vi "继保.vi"() -> ()   [LabVIEW 2015]
uses:
  <vilib>/Modbus/master/Modbus Master.lvclass
  <userlib>/QMH/Message Queue/Support/Enqueue Message (Single).vi
  Global control/global-2.vi
  <vilib>/Modbus/master/Create Master Instance (TCP).vi
  <userlib>/QMH/User Event - Stop/User Event - Stop.lvlib
  <userlib>/QMH/Message Queue/Message Queue.lvlib
panel:
  out "开入":T1
  out "软压板R":T2 caption="继保遥信"
  out "动作报告":T3
  out "虚遥信":T4
  in  "软压板W":T2 caption="继保遥信"
  in  "遥控1合":bool
  in  "遥控1分":bool
  out "遥控R":bool[](array[boolean])
  in  "HostThread":variant
  in  "Exit":bool
  out "遥测":u32[](array[numeric])
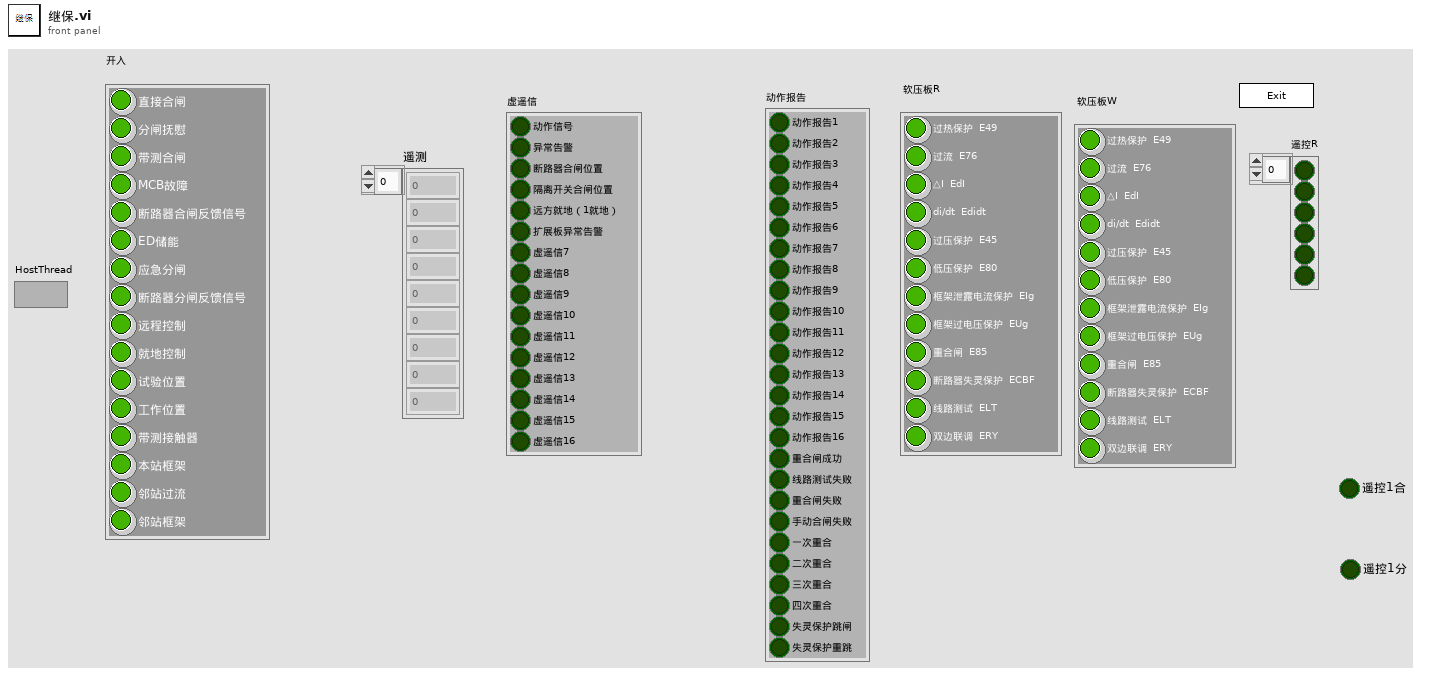
[diagram p1: front panel]
types:
  T1 = cluster{"直接合闸":bool, "分闸抚慰":bool, "带测合闸":bool, "MCB故障":bool, "断路器合闸反馈信号":bool, "ED储能":bool, "应急分闸":bool, "断路器分闸反馈信号":bool, "远程控制":bool, "就地控制":bool, "试验位置":bool, "工作位置":bool, "带测接触器":bool, "本站框架":bool, "邻站过流":bool, "邻站框架":bool}
  T2 = cluster{"过热保护  E49":bool, "过流  E76":bool, "△I  EdI":bool, "di/dt  Edidt":bool, "过压保护  E45":bool, "低压保护  E80":bool, "框架泄露电流保护  EIg":bool, "框架过电压保护  EUg":bool, "重合闸  E85":bool, "断路器失灵保护  ECBF":bool, "线路测试  ELT":bool, "双边联调  ERY":bool}
  T3 = cluster{"动作报告1":bool, "动作报告2":bool, "动作报告3":bool, "动作报告4":bool, "动作报告5":bool, "动作报告6":bool, "动作报告7":bool, "动作报告8":bool, "动作报告9":bool, "动作报告10":bool, "动作报告11":bool, "动作报告12":bool, "动作报告13":bool, "动作报告14":bool, "动作报告15":bool, "动作报告16":bool, "重合闸成功":bool, "线路测试失败":bool, "重合闸失败":bool, "手动合闸失败":bool, "一次重合":bool, "二次重合":bool, "三次重合":bool, "四次重合":bool, "失灵保护跳闸":bool, "失灵保护重跳":bool}
  T4 = cluster{"动作信号":bool, "异常告警":bool, "断路器合闸位置":bool, "隔离开关合闸位置":bool, "远方就地（1就地）":bool, "扩展板异常告警":bool, "虚遥信7":bool, "虚遥信8":bool, "虚遥信9":bool, "虚遥信10":bool, "虚遥信11":bool, "虚遥信12":bool, "虚遥信13":bool, "虚遥信14":bool, "虚遥信15":bool, "虚遥信16":bool}
  T5 = cluster{"Controls":cluster{"Exit":refnum<vi>}, "Thread":cluster{"ThisQ":string, "ThisVI":refnum<vi>, "HostQ":string, "HostRef":refnum<vi>, "SlavesQ":string[], "SlavesRef":refnum<vi>[]}, "Data":cluster{"Replace":bool}, "User":cluster{"Name":string}, "TCP master instance":refnum<class "Modbus Master.lvclass">}
  T6 = cluster{"开入1":bool, "开入2":bool, "开入3":bool, "开入4":bool, "开入5":bool, "开入6":bool, "开入7":bool, "开入8":bool, "开入9":bool, "开入10":bool, "开入11":bool, "开入12":bool, "开入13":bool, "开入14":bool, "开入15":bool, "开入16":bool}
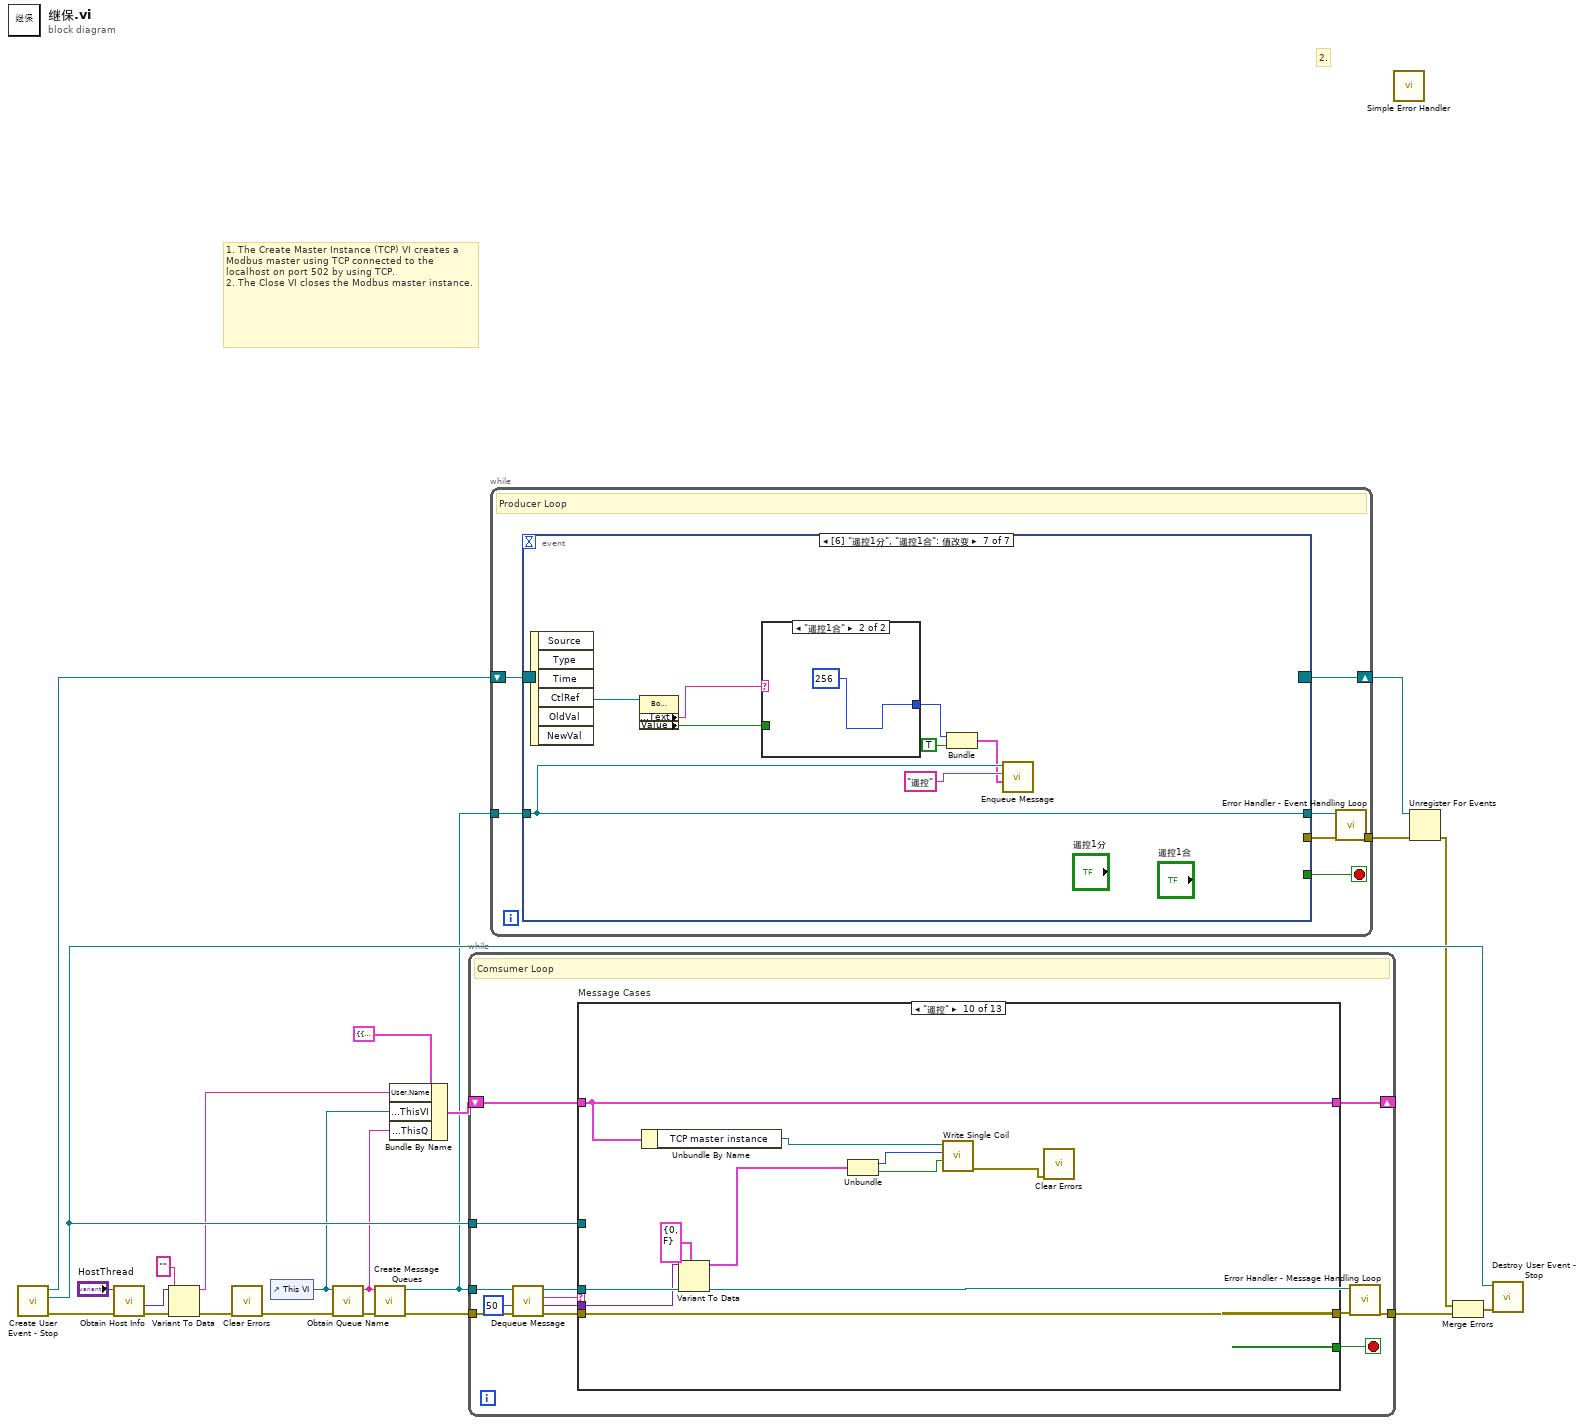
[diagram p0: block diagram]
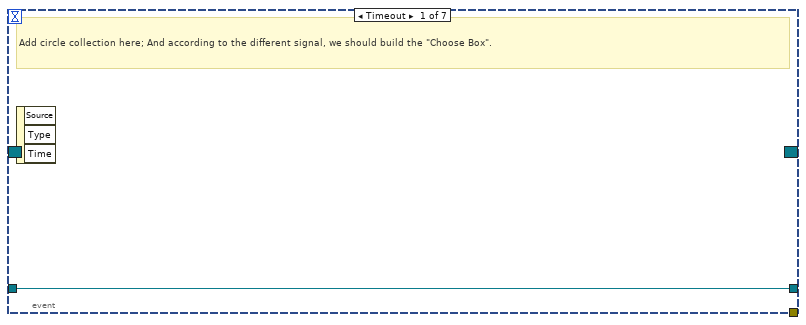
[diagram p2: hidden frame]
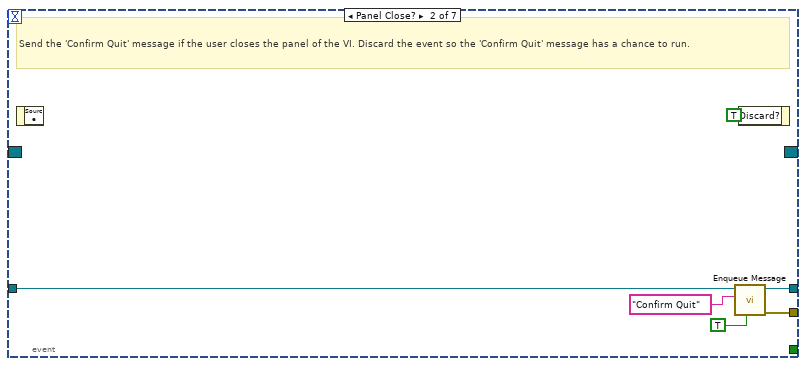
[diagram p3: hidden frame]
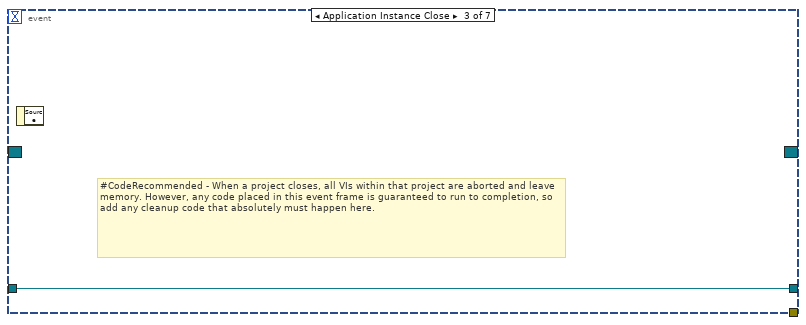
[diagram p4: hidden frame]
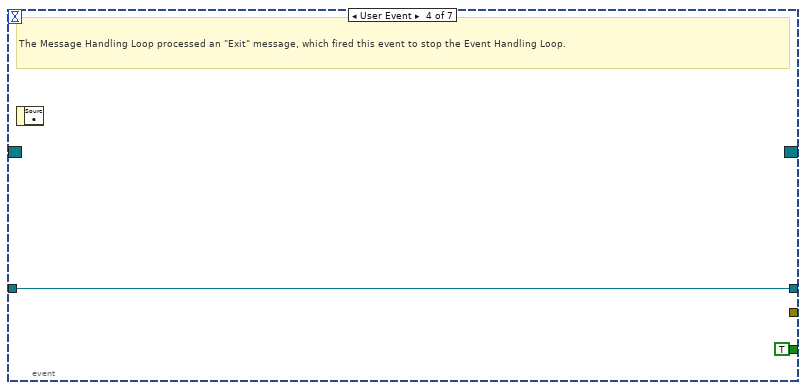
[diagram p5: hidden frame]
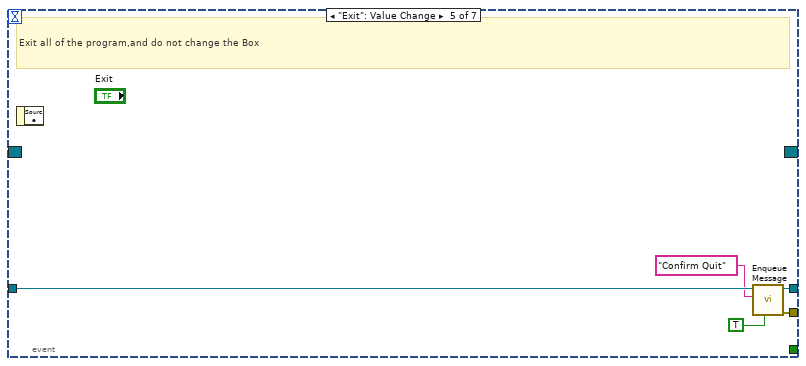
[diagram p6: hidden frame]
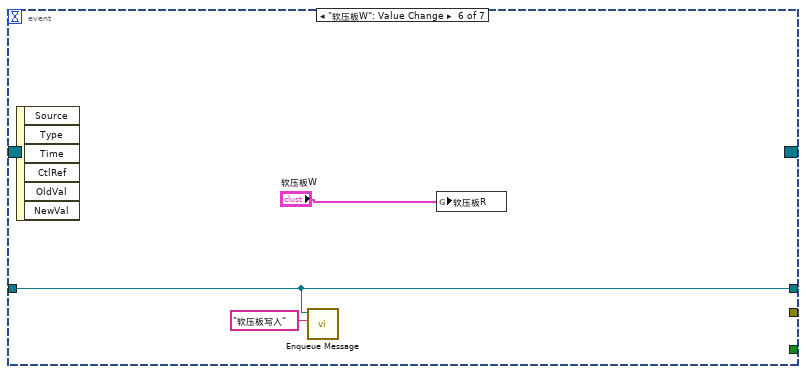
[diagram p7: hidden frame]
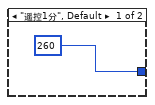
[diagram p8: hidden frame]
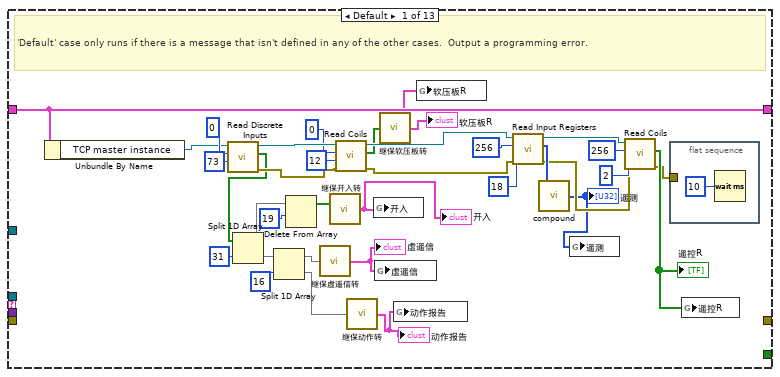
[diagram p9: hidden frame]
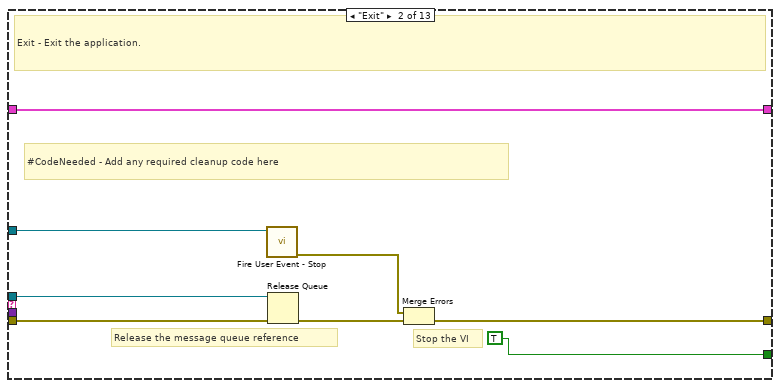
[diagram p10: hidden frame]
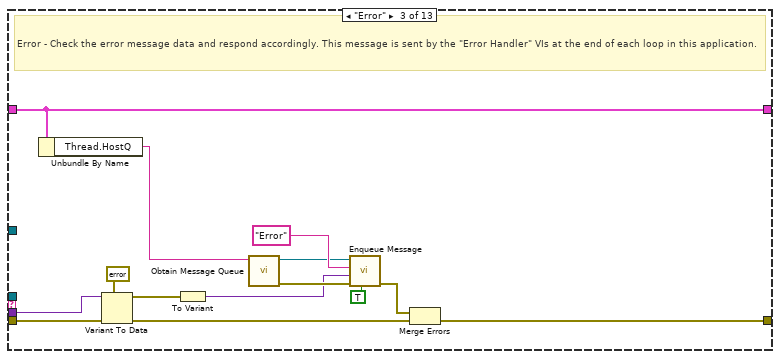
[diagram p11: hidden frame]
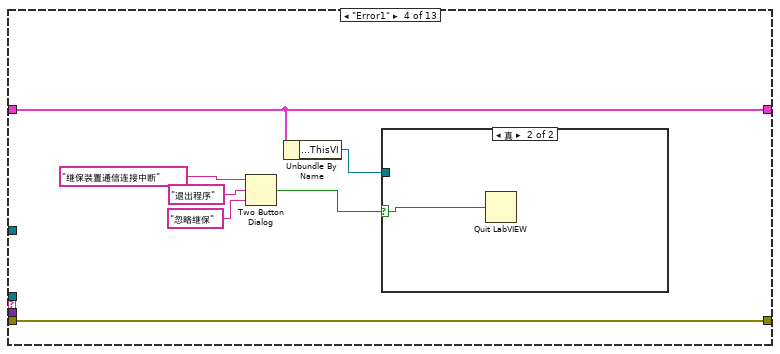
[diagram p12: hidden frame]
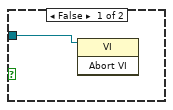
[diagram p13: hidden frame]
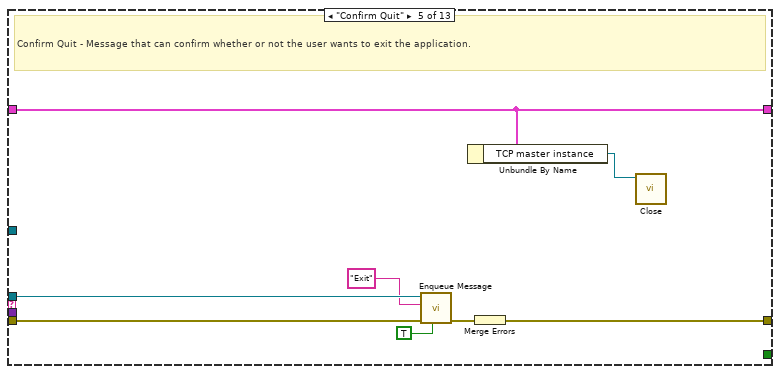
[diagram p14: hidden frame]
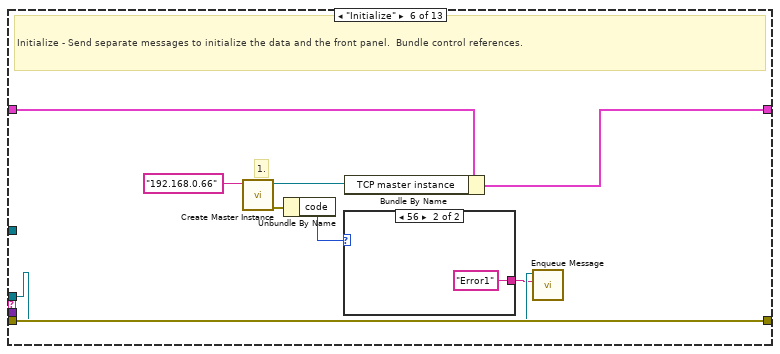
[diagram p15: hidden frame]
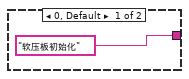
[diagram p16: hidden frame]
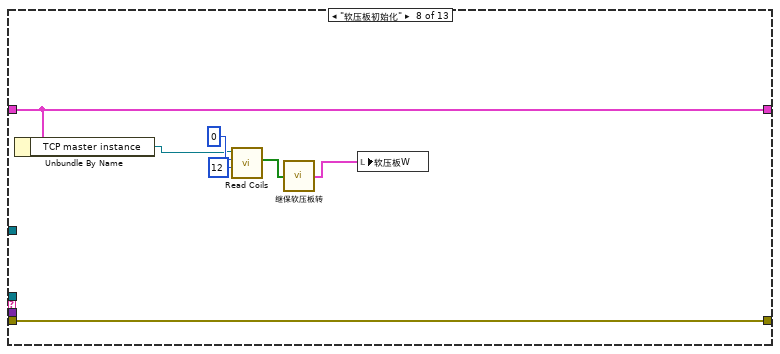
[diagram p18: hidden frame]
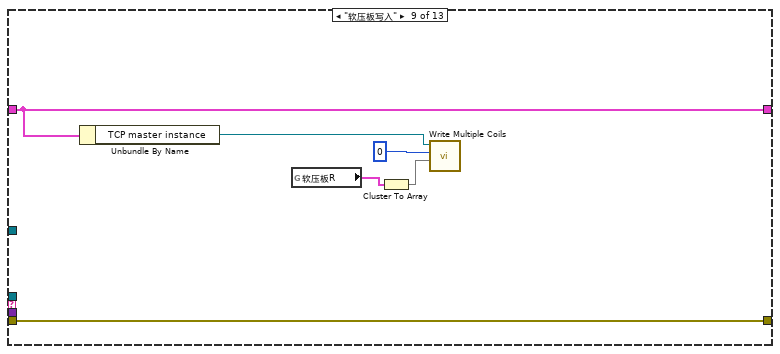
[diagram p19: hidden frame]
diagram:
  # "2."
  # "1. The Create Master Instance (TCP) VI creates a Modbus master using TCP connected to the localhost on port 502 by using TCP.\n2. The Close VI closes the Modbus master instance."
  n1 = call <userlib>:"Create User Event - Stop.vi"() -> ("error out"=w9:errorcluster, "User Event - Stop"=w18:refnum<user-event>, "Stop Event Registration Refnum"=w20:refnum<event-registration>)  [unwired: 9 in]
  n2 = call <userlib>:"Obtain Host Info.vi"("error in (no error)"=w9, "HostThread"="HostThread") -> ("error out"=w6:errorcluster, "Data"=w5:variant)  [unwired: 6 in, 2 out]
  n3 = Variant To Data(error in=w6, type="", Variant=w5) -> (data=w1:string, error out=w3:errorcluster)
  n4 = call <vilib>:"Clear Errors.vi"("error in (no error)"=w3) -> ("error out"=w2:errorcluster)  [unwired: 5 in, 1 out]
  n5 = control-ref of="This VI"() -> (w11:refnum<vi>)
  n6 = call <userlib>:"Obtain Queue Name.vi"("error in (no error)"=w2, "VI Refnum"=w11) -> ("error out"=w14:errorcluster, "ViName"=w10:string)  [unwired: 8 in]
  n7 = call <userlib>:"Create Message Queues.vi"("error in (no error)"=w14, "name (unnamed)"=w10) -> ("error out"=w22:errorcluster, "QueueHandler"=w7:refnum<queue>)  [unwired: 8 in]
  n8 = Bundle By Name(cluster=T5 {"Controls"={"Exit"=refnum}, "Thread"={"ThisQ"="", "ThisVI"=refnum, "HostQ"="", "HostRef"=refnum, "SlavesQ"=[], "SlavesRef"=[]}, "Data"={"Replace"=FALSE}, "User"={"Name"=""}, "TCP master instance"=refnum} ("Data Cluster"), "User.Name"=w1, "Thread.ThisVI"=w11, "Thread.ThisQ"=w10) -> (w12:T5)
  n9 = while {
    tunnel: w7 -> [w27]
    shift-right: [w34] -> _
    shift-left: w12 -> [w35]
    tunnel: w18 -> [w32]
    tunnel: w22 -> [w31]
    tunnel: [w25] -> w21
    stop <- w33 stop-if-true
    # "Comsumer Loop"
    n10 = call <userlib>:"Dequeue Message.vi"("error in (no error)"=w31, "timeout in ms (-1)"=50, "Message Queue"=w27) -> ("error out"=w30:errorcluster, "Message Data"=w28:variant, "Message"=w29:string, "dup Message Queue"=w26:refnum<queue>)  [unwired: 5 in]
    n11 = case "Message Cases" shown="\"遥控\"" w29 {
      tunnel: w26 -> [_ w78 _ _ w106 w111 _ _ _ _ _ _ _]
      tunnel: w30 -> [_ w73 w92 w99 w109 w118 w122 w129 w135 w144 w146 w147 w150]
      tunnel: [_ w74 w87 w99 w108 w118 w122 w129 w135 w144 w146 w147 w150] -> w24
      tunnel: w35 -> [w58 w77 w84 w94 w103 w116 w121 w126 w134 w143 w145 w148 w149]
      tunnel: [w58 w77 w84 w94 w103 w115 w121 w126 w134 w143 w145 w148 w149] -> w34
      tunnel: [_ TRUE _ _ _ _ _ _ _ _ _ _ _] -> w33
      tunnel: w28 -> [_ _ w91 _ _ _ _ _ _ w141 _ _ _]
      tunnel: w32 -> [_ w72 _ _ _ _ _ _ _ _ _ _ _]
      frame Default {
        # "'Default' case only runs if there is a message that isn't defined in any of the other cases.  Output a programming error."
        n12 = Unbundle By Name(w58) -> ("TCP master instance"=w57:refnum<class "Modbus Master.lvclass">)
        n13 = call-dynamic "Read Discrete Inputs.vi"("number of discrete inputs"=u16 73, "starting address"=u16 0, "Modbus master in"=w57) -> ("error out"=w65:errorcluster, "discrete input values"=w56:bool[], "Modbus master out"=w66:refnum<class "Modbus Master.lvclass">)  [unwired: 6 in]
        n14 = Split 1D Array(array=w56, index=31 ("索引")) -> (first subarray=w47:bool[], second subarray=w54:bool[])
        n15 = Split 1D Array(array=w54, index=16 ("索引")) -> (first subarray=w44:bool[], second subarray=w43:bool[])
        n16 = Delete From Array(array=w47, length=19 ("长度")) -> (array with subset deleted=w45:bool[])  [unwired: 1 in, 1 out]
        n17 = call "继保虚遥信转.vi"("虚遥信"=w44) -> ("虚遥信out"=w41:T4)
        "虚遥信" <- w41
        n18 = call "继保开入转.vi"("开入"=w45) -> ("开入out"=w38:T6)
        "开入" <- w38
        n19 = call-dynamic "Read Coils.vi"("error in (no error)"=w65, "number of coils"=u16 12, "starting address"=u16 0, "Modbus master in"=w66) -> ("error out"=w63:errorcluster, "coil values"=w42:bool[], "Modbus master out"=w64:refnum<class "Modbus Master.lvclass">)  [unwired: 5 in]
        n20 = call "继保动作转.vi"("动作报告in"=w43) -> ("动作报告out"=w40:T3)
        "动作报告" <- w40
        n21 = global write "global-2.vi" "开入"(w38) -> ()
        n22 = global write "global-2.vi" "虚遥信"(w41) -> ()
        n23 = call "继保软压板转.vi"("软压板Rin"=w42) -> ("软压板Rout"=w39:T2)
        "软压板R" <- w39
        n24 = global write "global-2.vi" "动作报告"(w40) -> ()
        n25 = global write "global-2.vi" "软压板R"(w39) -> ()
        n26 = call-dynamic "Read Input Registers.vi"("error in (no error)"=w63, "number of input registers"=u16 18 ("number of discrete inputs"), "starting address"=u16 256, "Modbus master in"=w64) -> ("error out"=w46:errorcluster, "register values"=w68:u16[], "Modbus master out"=w52:refnum<class "Modbus Master.lvclass">)  [unwired: 5 in]
        n27 = call "compound.vi"("In Array"=w68) -> ("Result"=w37:u32[])
        "遥测" <- w37
        n28 = global write "global-2.vi" "遥测"(w37) -> ()
        n29 = call-dynamic "Read Coils.vi"("error in (no error)"=w46, "number of coils"=u16 2, "starting address"=u16 256, "Modbus master in"=w52) -> ("error out"=w36:errorcluster, "coil values"=w49:bool[])  [unwired: 5 in, 1 out]
        "遥控R" <- w49
        n30 = flat-sequence {
          tunnel: w36 -> [_]
          frame #0 {
            n31 = Wait (ms)(milliseconds to wait=u32 10 ("等待时间（毫秒）")) -> ()  [unwired: 1 out]
          }
        }
        n32 = global write "global-2.vi" "遥控R"(w49) -> ()
      }
      frame "Exit" {
        # "Stop the VI"
        # "Release the message queue reference"
        # "#CodeNeeded - Add any required cleanup code here"
        # "Exit - Exit the application."
        n33 = call <userlib>:"Fire User Event - Stop.vi"("User Event - Stop"=w72) -> ("error out"=w71:errorcluster)  [unwired: 10 in]
        n34 = Release Queue(queue=w78, error in (no error)=w73) -> (error out=w75:errorcluster)  [unwired: 1 in, 2 out]
        n35 = Merge Errors(w71, w75) -> (w74:errorcluster)
      }
      frame "Error" {
        # "Error - Check the error message data and respond accordingly. This message is sent by the \"Error Handler\" VIs at the end of each loop in this application."
        n36 = Unbundle By Name(w84) -> ("Thread.HostQ"=w83:string)
        n37 = Variant To Data(error in=w92, type=errorcluster {"status"=FALSE, "code"=0, "source"=""} ("error constant"), Variant=w91) -> (data=w80:errorcluster, error out=w89:errorcluster)
        n38 = To Variant(anything=w80) -> (Variant=w79:variant)
        n39 = call <userlib>:"Obtain Message Queue.vi"("name (unnamed)"=w83) -> ("error out"=w82:errorcluster, "Message Queue"=w81:refnum<queue>)  [unwired: 9 in]
        n40 = call-poly <userlib>:"Enqueue Message.vi"("Priority Message? (F)"=TRUE, "error in (no error)"=w82, "Message Data"=w79, "Message"="Error", "Message Queue"=w81) -> ("error out"=w88:errorcluster)  [unwired: 5 in, 1 out]
        n41 = Merge Errors(w88, w89) -> (w87:errorcluster)
      }
      frame "Error1" {
        n42 = Two Button Dialog(message="继保装置通信连接中断" ("消息"), 1:"忽略继保" ("F按钮名称（“取消”）"), 2:"退出程序" ("T按钮名称（“确定”）")) -> (T button?=w95:bool)
        n43 = Unbundle By Name(w94) -> ("Thread.ThisVI"=w93:refnum<vi>)
        n44 = case shown="真" w95 {
          selector: w95 -> [_ w101]
          tunnel: w93 -> [w100 _]
          frame False {
            n45 = invoke class="VI" method="Abort VI"(reference=w100) -> ()  [unwired: 2 in, 3 out]
          }
          frame True {
            n46 = Quit LabVIEW(quit? (T)=w101) -> ()
          }
        }
      }
      frame "Confirm Quit" {
        # "Confirm Quit - Message that can confirm whether or not the user wants to exit the application."
        n47 = call-poly <userlib>:"Enqueue Message.vi"("Priority Message? (F)"=TRUE, "error in (no error)"=w109, "Message"="Exit", "Message Queue"=w106) -> ("error out"=w107:errorcluster)  [unwired: 6 in, 1 out]
        n48 = Unbundle By Name(w103) -> ("TCP master instance"=w102:refnum<class "Modbus Master.lvclass">)
        n49 = Merge Errors(w107) -> (w108:errorcluster)
        n50 = call-dynamic "Close.vi"("Modbus master in"=w102) -> ()  [unwired: 10 in, 1 out]
      }
      frame "Initialize" {
        # "1."
        # "Initialize - Send separate messages to initialize the data and the front panel.  Bundle control references."
        n51 = call-poly <vilib>:"Create Master Instance.vi"("address"="192.168.0.66") -> ("error out"=w113:errorcluster, "TCP master instance"=w114:refnum<class "Modbus Master.lvclass">)  [unwired: 9 in]
        n52 = Unbundle By Name(w113) -> ("code"=w112:i32)
        n53 = case shown="56" w112 {
          tunnel: ["软压板初始化" ("Message") "Error1" ("Message")] -> w110
          frame 0, Default {
          }
          frame 56 {
          }
        }
        n54 = Bundle By Name(cluster=w116, "TCP master instance"=w114) -> (w115:T5)
        n55 = call-poly <userlib>:"Enqueue Message.vi"("Message"=w110, "Message Queue"=w111) -> ()  [unwired: 8 in, 2 out]
      }
      frame "<-------UI-------->" {
      }
      frame "软压板初始化" {
        n56 = Unbundle By Name(w126) -> ("TCP master instance"=w125:refnum<class "Modbus Master.lvclass">)
        n57 = call-dynamic "Read Coils.vi"("number of coils"=u16 12, "starting address"=u16 0, "Modbus master in"=w125) -> ("coil values"=w124:bool[])  [unwired: 6 in, 2 out]
        n58 = call "继保软压板转.vi"("软压板Rin"=w124) -> ("软压板Rout"=w123:T2)
        n59 = local write "软压板W"(w123) -> ()
      }
      frame "软压板写入" {
        n60 = Unbundle By Name(w134) -> ("TCP master instance"=w133:refnum<class "Modbus Master.lvclass">)
        n61 = global read "global-2.vi" "软压板R"() -> (w131:T2)
        n62 = Cluster To Array(cluster=w131) -> (array=w130:bool[])
        n63 = call-dynamic "Write Multiple Coils.vi"("coil values"=w130, "starting address"=u16 0, "Modbus master in"=w133) -> ()  [unwired: 7 in, 2 out]
      }
      frame "遥控" {
        n64 = Unbundle By Name(w143) -> ("TCP master instance"=w142:refnum<class "Modbus Master.lvclass">)
        n65 = Variant To Data(type=cluster{u16, "Value":bool} {0, "Value"=FALSE} ("输出簇"), Variant=w141) -> (data=w139:cluster{u16, "Value":bool})  [unwired: 1 in, 1 out]
        n66 = Unbundle(w139) -> (w136:u16, "Value"=w138:bool)
        n67 = call-dynamic "Write Single Coil.vi"("coil value"=w138, "address"=w136, "Modbus master in"=w142) -> ("error out"=w137:errorcluster)  [unwired: 7 in, 1 out]
        n68 = call <vilib>:"Clear Errors.vi"("error in (no error)"=w137) -> ()  [unwired: 5 in, 2 out]
      }
      frame "<------Core------>" {
      }
      frame "Core_InitializeRef" {
        # "Initialize control references. For there is not enough space to locate all the control references, separate the codes into 2 messages"
      }
      frame "<---Operation--->" {
      }
    }
    n69 = call <userlib>:"Error Handler - Message Handling Loop.vi"("error in (no error)"=w24, "Message Queue"=w26) -> ("dup error in"=w25:errorcluster)  [unwired: 8 in, 1 out]
  }
  n70 = while {
    tunnel: w7 -> [w157]
    shift-right: [w155] -> w16
    shift-left: w20 -> [w156]
    tunnel: [w151] -> w15
    stop <- w153 stop-if-true
    # "Producer Loop"
    n71 = event shown="[6] \"遥控1分\", \"遥控1合\": 值改变" {
      selector: w156 -> [_ _ _ _ _ _ _]
      dyn-events: [_ _ _ _ _ _ _] -> w155
      timeout: _ -> [_ _ _ _ _ _ _]
      tunnel: [_ _ _ TRUE ("Discard?") _ _ _] -> w153
      tunnel: w157 -> [w158 w163 w165 w167 w172 w175 w181]
      tunnel: [_ w162 _ _ w170 _ _] -> w154
      tunnel: [w158 w161 w165 w167 w171 w175 w181] -> w152
      event Timeout {
        # "Add circle collection here; And according to the different signal, we should build the \"Choose Box\"."
        n72 = event-data() -> ()  [unwired: 1 in, 3 out]
      }
      event Panel Close? {
        # "Send the 'Confirm Quit' message if the user closes the panel of the VI. Discard the event so the 'Confirm Quit' message has a chance to run."
        n73 = event-data() -> ()  [unwired: 1 in, 1 out]
        n74 = call-poly <userlib>:"Enqueue Message.vi"("Priority Message? (F)"=TRUE, "Message"="Confirm Quit", "Message Queue"=w163) -> ("error out"=w162:errorcluster, "dup Message Queue"=w161:refnum<queue>)  [unwired: 7 in]
        n75 = event-data("Discard?"=TRUE) -> ()  [unwired: 1 in, 1 out]
      }
      event Application Instance Close {
        # "#CodeRecommended - When a project closes, all VIs within that project are aborted and leave memory. However, any code placed in this event frame is guaranteed to run to completion, so add any cleanup code that absolutely must happen here."
        n76 = event-data() -> ()  [unwired: 1 in, 1 out]
      }
      event User Event {
        # "The Message Handling Loop processed an \"Exit\" message, which fired this event to stop the Event Handling Loop."
        n77 = event-data() -> ()  [unwired: 1 in, 1 out]
      }
      event "Exit": Value Change {
        # "Exit all of the program,and do not change the Box"
        n78 = event-data() -> ()  [unwired: 1 in, 1 out]
        n79 = call-poly <userlib>:"Enqueue Message.vi"("Priority Message? (F)"=TRUE, "Message"="Confirm Quit", "Message Queue"=w172) -> ("error out"=w170:errorcluster, "dup Message Queue"=w171:refnum<queue>)  [unwired: 7 in]
      }
      event "软压板W": Value Change {
        n80 = event-data() -> ()  [unwired: 1 in, 6 out]
        n81 = call-poly <userlib>:"Enqueue Message.vi"("Message"="软压板写入", "Message Queue"=w175) -> ()  [unwired: 8 in, 2 out]
        n82 = global write "global-2.vi" "软压板R"("软压板W") -> ()
      }
      event "遥控1分", "遥控1合": Value Change {
        n83 = event-data() -> ("CtlRef"=w183:refnum<vi>)  [unwired: 1 in, 5 out]
        n84 = property class="Bool (严格)"(reference=w183) -> ("Label.Text"=w182:string, "Value"=w179:bool)  [unwired: 1 in, 2 out]
        n85 = case shown="\"遥控1合\"" w182 {
          tunnel: w179 -> [_ _]
          tunnel: [u16 260 u16 256] -> w178
          frame "遥控1分", Default {
          }
          frame "遥控1合" {
          }
        }
        n86 = Bundle(w178, TRUE) -> (w177:cluster{u16, bool})  [unwired: 1 in]
        n87 = call-poly <userlib>:"Enqueue Message.vi"("Message Data"=w177, "Message"="遥控", "Message Queue"=w181) -> ()  [unwired: 7 in, 2 out]
      }
    }
    n88 = call <userlib>:"Error Handler - Event Handling Loop.vi"("error in (no error)"=w154, "Message Queue"=w152) -> ("dup error in"=w151:errorcluster)  [unwired: 8 in, 1 out]
  }
  n89 = call <vilib>:"Simple Error Handler.vi"() -> ()  [unwired: 5 in, 5 out]
  n90 = Unregister For Events(event registration refnum=w16, error in=w15) -> (error out=w17:errorcluster)
  n91 = Merge Errors(w17, w21) -> (w19:errorcluster)
  n92 = call <userlib>:"Destroy User Event - Stop.vi"("error in (no error)"=w19, "User Event - Stop"=w18) -> ()  [unwired: 9 in, 1 out]
